vi "populate_io_index_array.vi"(8 "error in (no error)":errorcluster, 11 "IO_variables_per_module":T1) -> (0 "error out":errorcluster, 2 "use_scanned_method":bool, 3 "IO_table_index_ordered":i32[](array[numeric]))   [LabVIEW 2015, in "Scan Engine runtime.lvclass"]
uses:
  Scan Engine runtime.lvclass
  Custom Ctrls/IO_index_map.ctl
  <vilib>/NI/Tag Bus/tag/Data Type.ctl
  Custom Ctrls/Index Map.ctl
  <resource>/objmgr/ni.var.rc
  <vilib>/NI/Tag Bus/tag/tag descriptor.lvclass
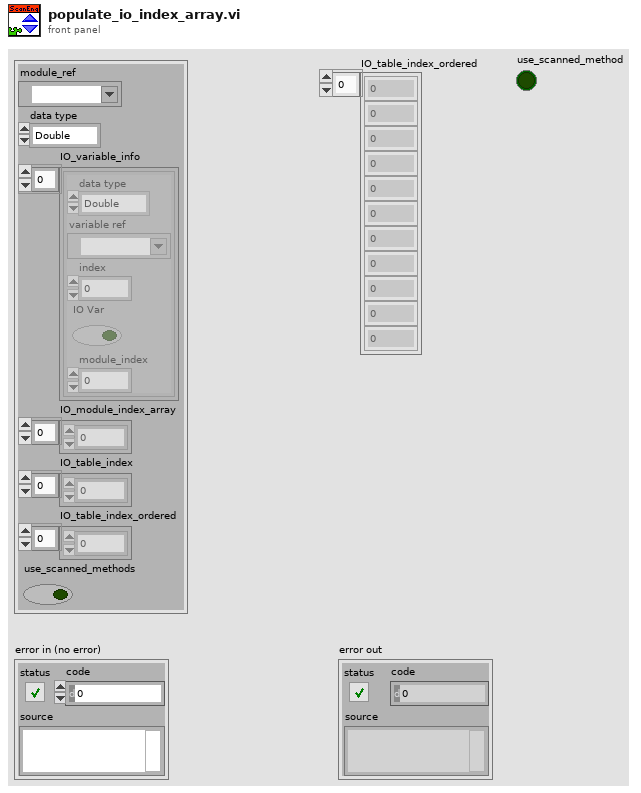
[diagram p1: front panel]
types:
  T1 = typedef "Scan Engine runtime.lvclass/IO_index_map.ctl" = cluster{"module_ref":refnum<k21>, "data type":T2, "IO_variable_info":T3[], "IO_module_index_array":i32[], "IO_table_index":i32[], "IO_table_index_ordered":i32[], "use_scanned_methods":bool}
  T2 = typedef "tag bus.lvlib/tag descriptor.lvclass/Data Type.ctl" = enum16{"Double", "Single", "I64", "I32", "I16", "I8", "U64", "U32", "U16", "U8", "Boolean", "String", "Array of Double", "Array of Single", "Array of I64", "Array of I32", "Array of I16", "Array of I8", "Array of U64", "Array of U32", "Array of U16", "Array of U8", "Array of Boolean", "Array of String"}
  T3 = typedef "Scan Engine runtime.lvclass/Index Map.ctl" = cluster{"data type":T2, "variable ref":refnum<k21>, "index":i32, "IO Var":bool, "module_index":i32}
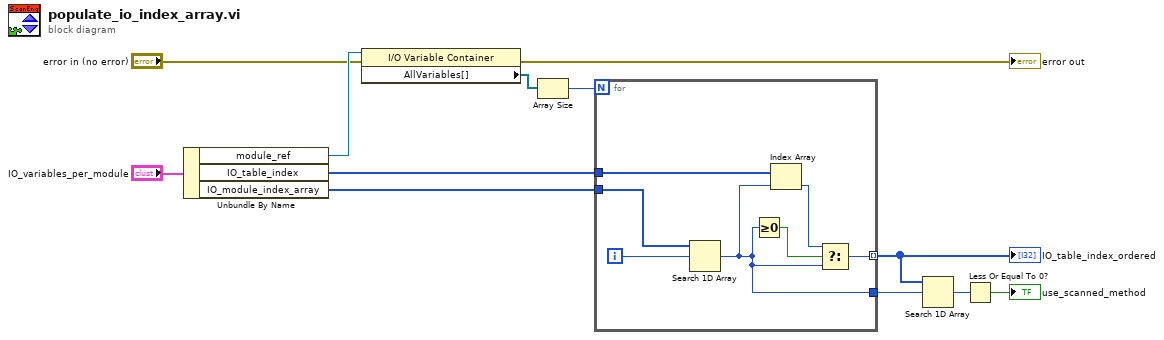
[diagram p0: block diagram]
diagram:
  n1 = Unbundle By Name("IO_variables_per_module") -> ("module_ref"=w7:refnum<k21>, "IO_table_index"=w10:i32[], "IO_module_index_array"=w11:i32[])
  n2 = property class="I/O Variable Container"(reference=w7, error in="error in (no error)") -> (error out=→"error out":errorcluster, "AllVariables[]"=w9:refnum<k21>[])  [unwired: 1 out]
  n3 = Array Size(array=w9) -> (size(s)=w8:i32)
  n4 = for {
    N: w8 -> [_]
    tunnel: w11 -> [w19]
    tunnel: w10 -> [w17]
    tunnel: [w15] -> w6 mode=indexing
    tunnel: [w13] -> w5
    i -> [w18]
    n5 = Search 1D Array(1D array=w19, element=w18) -> (index of element=w13:i32)  [unwired: 1 in]
    n6 = Greater Or Equal To 0?(x=w13) -> (x >= 0?=w14:bool)
    n7 = Index Array(array=w17, index=w13) -> (element=w16:i32)
    n8 = Select(t=w16, s=w14, f=w13) -> (s? t:f=w15:i32)
  }
  "IO_table_index_ordered" <- w6
  n9 = Search 1D Array(1D array=w6, element=w5) -> (index of element=w4:i32)  [unwired: 1 in]
  n10 = Less Or Equal To 0?(x=w4) -> (x <= 0?=→"use_scanned_method":bool)
